vi "Find Intensity Peaks.vi"(0 "Normalized Intensity Data":dbl[][](array[numeric]), 1 "Gaussian Fit Method":T1 items=["Least Square", "Least Absolute Residual", "Bisquare"], 2 "Intensity Threshold":i32, 3 "Index":i32, 4 "Peak Detector Width":i32=3 min=3) -> (5 "Array":cluster{"Locations":dbl[], "Amplitudes":dbl[]}[](array[cluster]))   [LabVIEW 2012]
uses:
  <vilib>/Analysis/6fits.llb/Curve Fitting Criteria.ctl
  <vilib>/Analysis/NI_AALPro.lvlib
  <vilib>/Analysis/NI_AAL_SigProc.lvlib
panel:
  out "standard deviation":dbl
  out "residue":dbl
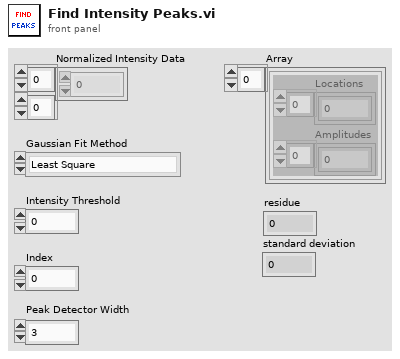
[diagram p1: front panel]
types:
  T1 = typedef "NI_AALPro.lvlib/Curve Fitting Criteria.ctl" = u16
  T2 = cluster{i32[], "Normalized Intensity Data":dbl[]}
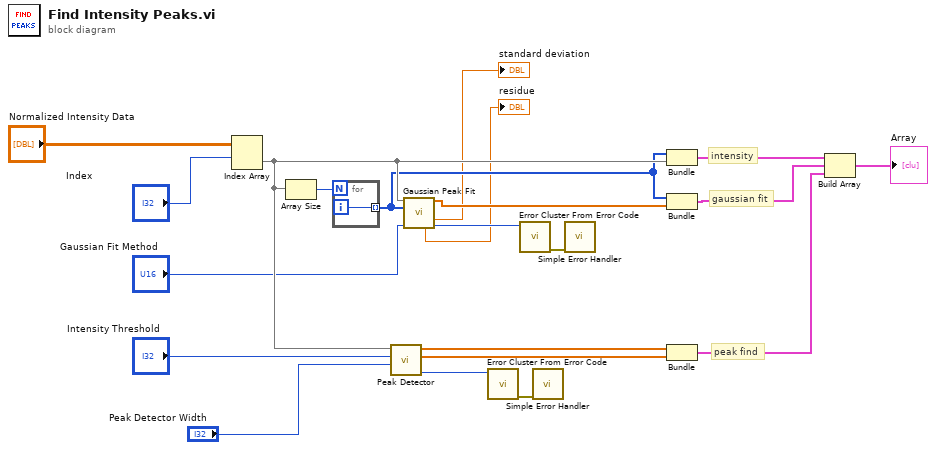
[diagram p0: block diagram]
diagram:
  # "peak find"
  # "gaussian fit"
  # "intensity"
  n1 = Index Array(array="Normalized Intensity Data", index (row)="Index") -> (element=w14:dbl[])  [unwired: 1 in]
  n2 = Array Size(array=w14) -> (size(s)=w8:i32)
  n3 = for {
    N: w8 -> [_]
    tunnel: [w22] -> w11 mode=indexing
    i -> [w22]
  }
  n4 = call <vilib>:"Peak Detector.vi"("width"="Peak Detector Width", "threshold"="Intensity Threshold", "X"=w14) -> ("error"=w1:i32, "Amplitudes"=w17:dbl[], "Locations"=w16:dbl[])  [unwired: 4 in, 2 out]
  n5 = call <vilib>:"Gaussian Peak Fit.vi"("Y"=w14, "X"=w11, "method"="Gaussian Fit Method") -> ("Best Gaussian Fit"=w12:dbl[], "standard deviation"=→"standard deviation":dbl, "residue"=→"residue":dbl, "error"=w20:i32)  [unwired: 6 in, 3 out]
  n6 = call <vilib>:"Error Cluster From Error Code.vi"("error code (0)"=w1) -> ("error out"=w2:errorcluster)  [unwired: 8 in]
  n7 = call <vilib>:"Error Cluster From Error Code.vi"("error code (0)"=w20) -> ("error out"=w21:errorcluster)  [unwired: 8 in]
  n8 = call <vilib>:"Simple Error Handler.vi"("error in (no error)"=w2) -> ()  [unwired: 4 in, 5 out]
  n9 = call <vilib>:"Simple Error Handler.vi"("error in (no error)"=w21) -> ()  [unwired: 4 in, 5 out]
  n10 = Bundle(w11, "Normalized Intensity Data"=w14) -> (w10:T2)  [unwired: 1 in]
  n11 = Bundle(w11, "Best Gaussian Fit"=w12) -> (w13:cluster{i32[], "Best Gaussian Fit":dbl[]})  [unwired: 1 in]
  n12 = Bundle("Locations"=w16, "Amplitudes"=w17) -> (w18:cluster{"Locations":dbl[], "Amplitudes":dbl[]})  [unwired: 1 in]
  n13 = Build Array(w10, w13, w18) -> (→"Array":cluster{"Locations":dbl[], "Amplitudes":dbl[]}[])
